vi "test_randn.vi"() -> ()   [LabVIEW 2019]
uses:
  <vilib>/ptbypt/NI_PtbyPt.lvlib
  <vilib>/Analysis/NI_AALBase.lvlib
panel:
  out "randn":cluster{dbl, "Gaussian white noise":dbl}(graph)
  in  "정지":bool
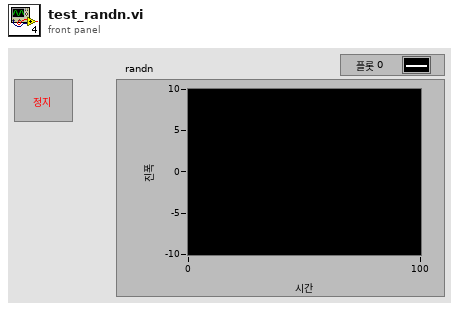
[diagram p1: front panel]
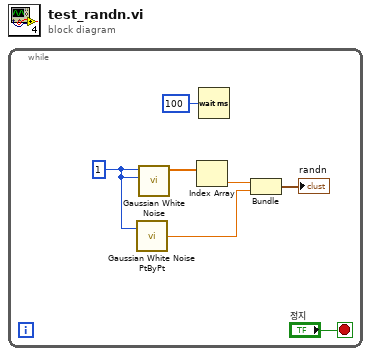
[diagram p0: block diagram]
diagram:
  n1 = while {
    stop <- "정지" stop-if-true
    w7 = 1 ("samples")
    n2 = call <vilib>:"Gaussian White Noise PtByPt.vi"("standard deviation"=w7) -> ("Gaussian white noise"=w6:dbl)  [unwired: 2 in]
    n3 = call <vilib>:"Gaussian White Noise.vi"("standard deviation"=w7, "samples"=w7) -> ("Gaussian noise pattern"=w5:dbl[])  [unwired: 8 in, 1 out]
    n4 = Index Array(array=w5) -> (element=w4:dbl)  [unwired: 1 in]
    n5 = Wait (ms)(milliseconds to wait=u32 100 ("대기 시간 (ms)")) -> ()  [unwired: 1 out]
    n6 = Bundle(w4, "Gaussian white noise"=w6) -> (→"randn":cluster{dbl, "Gaussian white noise":dbl})  [unwired: 1 in]
  }
